vi "Register MenuItem Callback.vi"(0 "NotifyIcon in":refnum<class "NotifyIcon.lvclass">, 7 "MenuItem":refnum<k24>, 11 "error in (no error)":errorcluster) -> (4 "NotifyIcon out":refnum<class "NotifyIcon.lvclass">, 8 "dub MenuItem":refnum<k24>, 15 "error out":errorcluster)   [LabVIEW 2017, in "NotifyIcon.lvclass"]
doc: "This VI registers the Click event callback VI for the Menu Item reference by the <b>MenuItem</b> input.\n\n\nStinus Olsen\nCIM Industrial Systems A/S\n22. Feb. 2011 15:05\nmailto: seo@cim.as"
uses:
  NotifyIcon.lvclass
  System.Windows.Forms
  NotifyIcon.lvclass/NotifyIcon.ctl
panel:
  # "This VI belongs to the NotifyIcon Toolset. \nA toolset that makes it easy to create, control and manipulate a notification icon in the notification area of the Windows taskbar.\nThe toolset requires Microsoft .NET framework 2.0\n\n\nNOTICE -- YOU MUST LEAVE THIS NOTICE IN PLACE.  PER THE TERMS OF THE LICENSE BELOW, YOU MAY SUBLICENSE THIS SOFTWARE \nIN ANY WAY THAT DOES NOT CONFLICT WITH THIS LICENSE.\n\n### BSD License (http://www.opensource.org/licenses/bsd-license.php) Begin ###\n \nCopyright (c) 2011, Stinus Olsen <seo@cim.as>\n\nAll rights reserved.\n\nRedistribution and use in source and binary forms, with or without modification, are permitted provided that the following conditions are met:\n\n    * Redistributions of source code must retain the above copyright notice, this list of conditions and the following disclaimer.\n    * Redistributions in binary form must reproduce the above copyright notice, this list of conditions and the following disclaimer in the \n       documentation and/or other materials provided with the distribution.\n    * Neither the name of CIM Industrial Systems nor the names of its contributors may be used to endorse or promote products derived \n       from this software without specific prior written permission.\n\nTHIS SOFTWARE IS PROVIDED BY THE COPYRIGHT HOLDERS AND CONTRIBUTORS \"AS IS\" AND ANY EXPRESS OR IMPLIED WARRANTIES, \nINCLUDING, BUT NOT LIMITED TO, THE IMPLIED WARRANTIES OF MERCHANTABILITY AND FITNESS FOR A PARTICULAR PURPOSE ARE \nDISCLAIMED. IN NO EVENT SHALL THE COPYRIGHT OWNER OR CONTRIBUTORS BE LIABLE FOR ANY DIRECT, INDIRECT, INCIDENTAL,\n SPECIAL, EXEMPLARY, OR CONSEQUENTIAL DAMAGES (INCLUDING, BUT NOT LIMITED TO, PROCUREMENT OF SUBSTITUTE GOODS OR \nSERVICES; LOSS OF USE, DATA, OR PROFITS; OR BUSINESS INTERRUPTION) HOWEVER CAUSED AND ON ANY THEORY OF LIABILITY, \nWHETHER IN CONTRACT, STRICT LIABILITY, OR TORT (INCLUDING NEGLIGENCE OR OTHERWISE) ARISING IN ANY WAY OUT OF THE USE \nOF THIS SOFTWARE, EVEN IF ADVISED OF THE POSSIBILITY OF SUCH DAMAGE.\n\n### BSD License End ###"
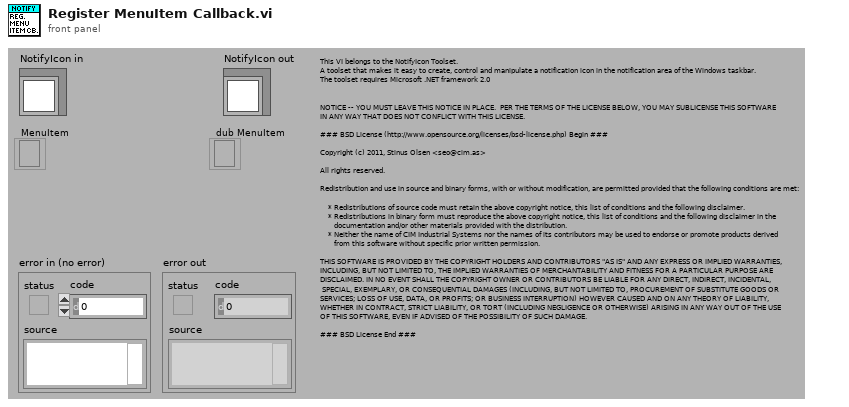
[diagram p1: front panel]
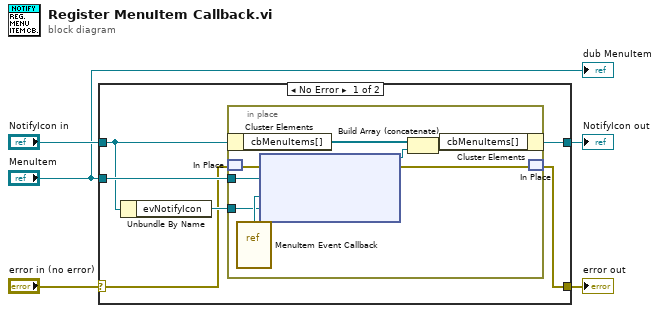
[diagram p0: block diagram]
diagram:
  n1 = case shown="No Error" "error in (no error)" {
    selector: "error in (no error)" -> [w7 w21]
    tunnel: [w6 w21] -> w4
    tunnel: [w8 w20] -> w2
    tunnel: "NotifyIcon in" -> [w9 w20]
    tunnel: "MenuItem" -> [w10 _]
    frame No Error {
      n2 = Unbundle By Name(w9) -> ("evNotifyIcon"=w11:refnum<user-event>)
      n3 = in-place {
        in-place-border: w11 -> [w13]
        in-place-border: w10 -> [w12]
        n4 = in-place-cluster #1(w9) -> ("cbMenuItems[]"=w18:refnum<k27>[])
        n5 = in-place-match #2(w7) -> (w15:errorcluster)
        n6 = vi-ref "MenuItem Event Callback.vi"() -> ("vi reference"=w19:refnum<vi>)
        n7 = node(w15, w12, w19, w13) -> (w16:refnum<k27>, w14:errorcluster)  [unwired: 1 in]
        n8 = Build Array (concatenate)(w18, w16) -> (w17:refnum<k27>[])
        n9 = in-place-cluster #1("cbMenuItems[]"=w17) -> (w8:refnum<class "NotifyIcon.lvclass">)
        n10 = in-place-match #2(w14) -> (w6:errorcluster)
      }
    }
    frame Error {
    }
  }
  "error out" <- w4
  "NotifyIcon out" <- w2
  "dub MenuItem" <- "MenuItem"
